vi "Launch Progress Bar.vi"(8 "error in (no error)":errorcluster, 9 "Enable Cancellation? (T)":bool=TRUE, 10 "Main Title (\"Working...\")":string="Working...", 11 "Total Count":i32) -> (0 "error out":errorcluster, 3 "Progress Bar Dialog":refnum<class "Progress Bar Dialog.lvclass">)   [LabVIEW 2017, in "Progress Bar Dialog.lvclass"]
doc: "Creates an instance of a progress bar dialog and sets the total number of steps that are expected to be performed. Note that the window will not appear until 500ms have passed in order to avoid rapidly flashing the window during repeated quick sequences."
uses:
  <vilib>/ProgressBar/Progress Bar Dialog.lvclass
  <vilib>/ProgressBar/Progress Bar Dialog.lvclass/Progress Bar Dialog.ctl
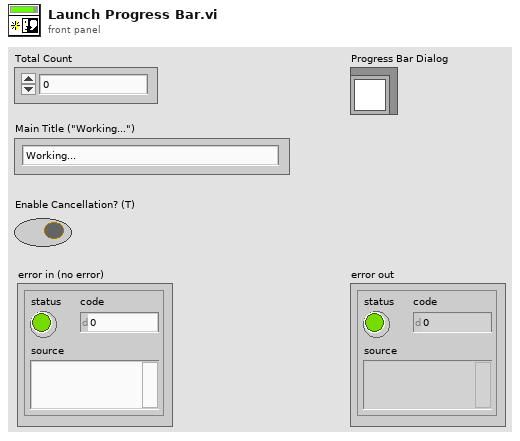
[diagram p1: front panel]
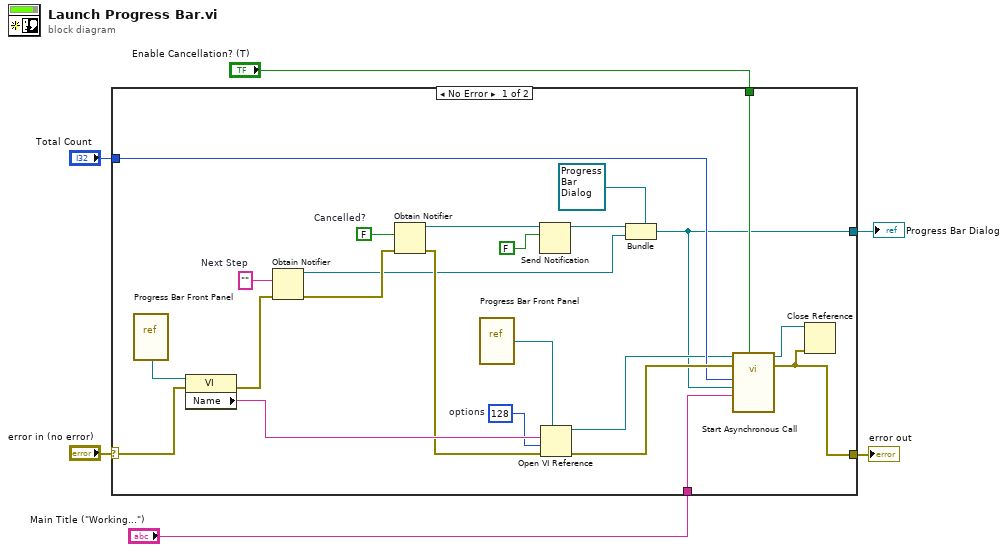
[diagram p0: block diagram]
diagram:
  n1 = case shown="No Error" "error in (no error)" {
    selector: "error in (no error)" -> [w24 w30]
    tunnel: [w7 w30] -> w6
    tunnel: "Total Count" -> [w25 _]
    tunnel: [w9 _] -> w3
    tunnel: "Main Title (\"Working...\")" -> [w12 _]
    tunnel: "Enable Cancellation? (T)" -> [w11 _]
    frame No Error {
      w16 = FALSE  # Cancelled?
      w23 = ""  # Next Step
      w26 = 128  # options
      n2 = vi-ref <vilib>:"Progress Bar Front Panel.vi"() -> (w27:refnum<vi>)
      n3 = property class="VI"(reference=w27, error in=w24) -> (error out=w22:errorcluster, "Name"=w28:string)  [unwired: 1 out]
      n4 = Obtain Notifier(notification data type=w23, error in (no error)=w22) -> (notifier out=w17:refnum<notifier>, error out=w19:errorcluster)  [unwired: 2 in, 1 out]
      n5 = Obtain Notifier(notification data type=w16, error in (no error)=w19) -> (notifier out=w14:refnum<notifier>, error out=w18:errorcluster)  [unwired: 2 in, 1 out]
      n6 = vi-ref <vilib>:"Progress Bar Front Panel.vi"() -> (w20:refnum<vi>)
      n7 = Send Notification(notification=FALSE, notifier=w14) -> (notifier out=w13:refnum<notifier>)  [unwired: 1 in, 1 out]
      n8 = Open VI Reference(type specifier VI Refnum (for type only)=w20, vi path=w28, options=w26, error in (no error)=w18) -> (vi reference=w21:refnum<vi>, error out=w29:errorcluster)  [unwired: 2 in]
      n9 = Bundle(cluster=refnum<class "Progress Bar Dialog.lvclass"> refnum ("Progress Bar Dialog"), w13, w17) -> (w9:refnum<class "Progress Bar Dialog.lvclass">)
      n10 = call-by-ref "Start Asynchronous Call"(reference=w21, error in=w29, "Enable Cancel?"=w11, "Main Title"=w12, "Progress Bar Dialog"=w9, "Total"=w25) -> (reference out=w8:refnum<vi>, error out=w7:errorcluster)  [unwired: 8 in]
      n11 = Close Reference(reference=w8, error in (no error)=w7) -> ()  [unwired: 1 out]
    }
    frame Error {
    }
  }
  "error out" <- w6
  "Progress Bar Dialog" <- w3
